vi "Reset_All_Relay.vi"(8 "error in (no error)":errorcluster caption="entrée d'erreur (pas d'erreur)", 11 "Class Relay_Board 16_Relay_R4D3D16 en entrée":refnum<class "Class Relay_Board 8_Relay_RY408D.lvclass">) -> (0 "error out":errorcluster caption="sortie d'erreur", 3 "Class Relay_Board 16_Relay_R4D3D16 en sortie":refnum<class "Class Relay_Board 8_Relay_RY408D.lvclass">)   [LabVIEW 2020, in "Library Instrument & Equipement.lvlib" / "Library Relay_Board.lvlib" / "Class Relay_Board 8_Relay_RY408D.lvclass"]
uses:
  Class Relay_Board 8_Relay_RY408D.lvclass
  Class Relay_Board 8_Relay_RY408D.lvclass/Class Relay_Board 8_Relay_RY408D.ctl
  Modbus/Modbus.lvclass
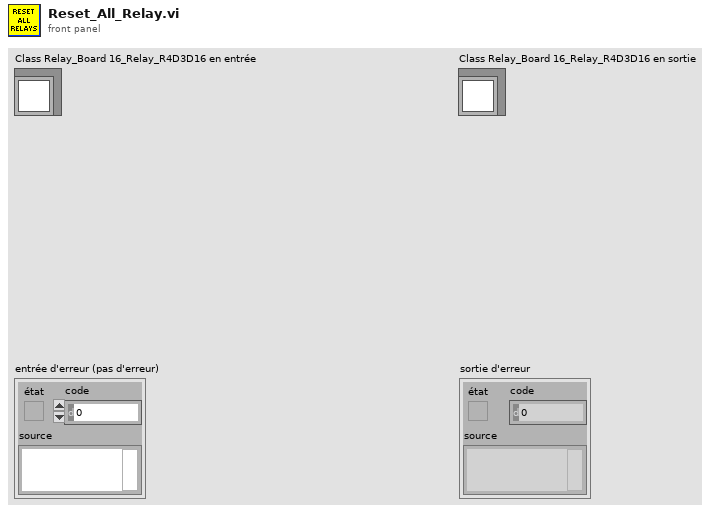
[diagram p1: front panel]
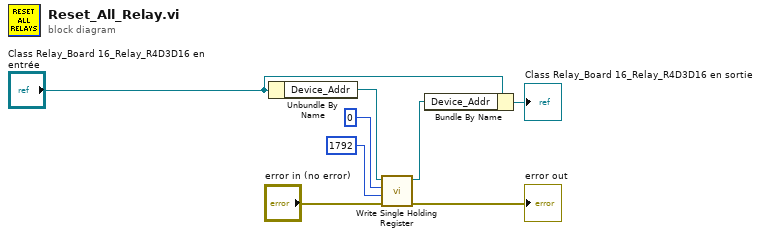
[diagram p0: block diagram]
diagram:
  n1 = Unbundle By Name("Class Relay_Board 16_Relay_R4D3D16 en entrée") -> ("Device_Addr"=w4:refnum<class "Modbus.lvclass">)
  n2 = call "Write Single Holding Register.vi"("error in (no error)"="error in (no error)", "value"=u16 1792, "address"=u16 0, "MODBUS in"=w4) -> ("error out"=→"error out":errorcluster, "MODBUS Out"=w5:refnum<class "Modbus.lvclass">)  [unwired: 6 in]
  n3 = Bundle By Name(cluster="Class Relay_Board 16_Relay_R4D3D16 en entrée", "Device_Addr"=w5) -> (→"Class Relay_Board 16_Relay_R4D3D16 en sortie":refnum<class "Class Relay_Board 8_Relay_RY408D.lvclass">)
